vi "TestRoomFGVRequests.vi"() -> (0 "error out":errorcluster, 2 "Pass":bool)   [LabVIEW 2015]
uses:
  TypeDef/RoomsActionEnum.ctl
  LVClasses/Flags/Flags.lvclass
  LVClasses/Room/Room.lvclass
panel:
  out "Add Request 2":string
  out "Read Request 2":string
  out "Remove Request":string
  out "Add Request 1":string
  out "Read Room 3":string
  out "Read Room 1":string
  out "Read Room 2":string
  out "Read Requests 1":string
  in  "FGV Room":i32=102
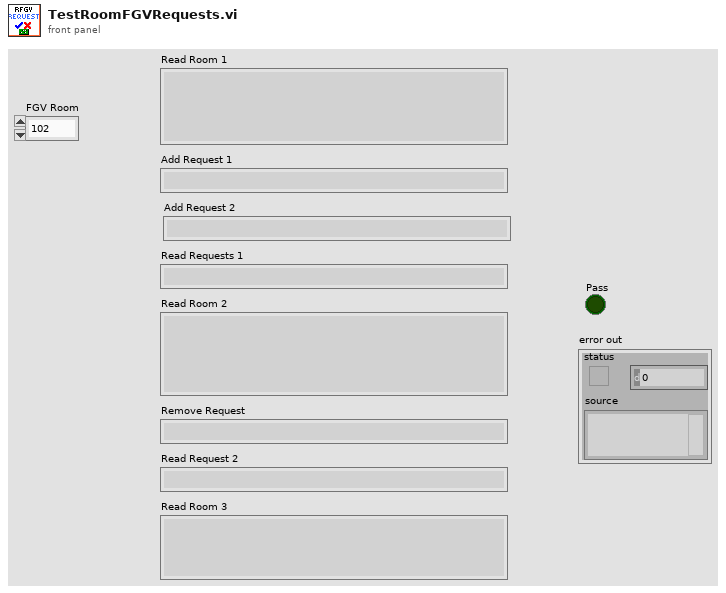
[diagram p1: front panel]
types:
  T1 = typedef "RoomsActionEnum.ctl" = enum16{"Init", "Add Room", "Remove Room", "Read Room", "Read Flag", "Read Flag State", "Write Flag State", "Read Flag Color", "Write Flag Color", "Read Bed Vacant", "Write Bed Vacant", "Read Personnel", "Add Personnel", "Remove Personnel", "Read Requests", "Add Request", "Remove Request", "Read Beacon ID", "Write Beacon ID", "Write Bed URL", "Read Bed URL", "Get Rooms Numbers"}
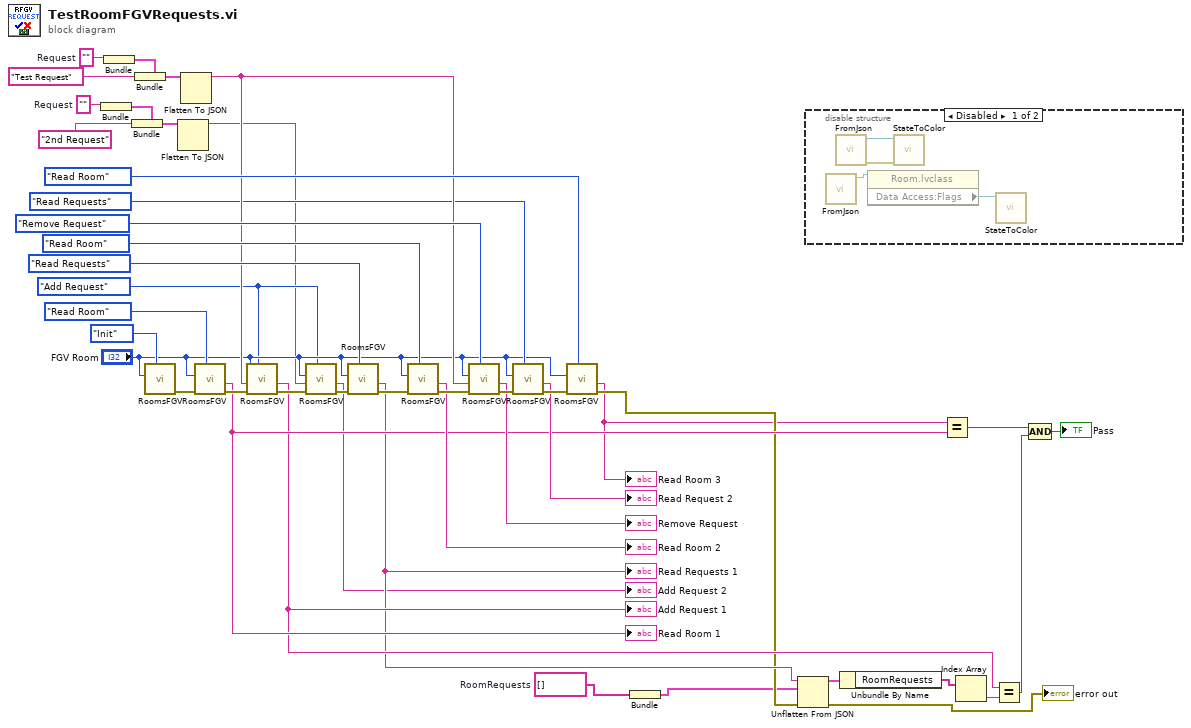
[diagram p0: block diagram]
diagram:
  w8 = ""  # Request
  w5 = string[] []  # RoomRequests
  w34 = ""  # Request
  w12 = RoomsActionEnum."Add Request"
  n1 = Bundle("Request"=w8) -> (w9:cluster{"Request":string})  [unwired: 1 in]
  n2 = Bundle("Request"=w34) -> (w33:cluster{"Request":string})  [unwired: 1 in]
  n3 = Bundle(cluster=w9, "Request"="2nd Request" ("Request 2")) -> (w10:cluster{"Request":string})
  n4 = Bundle(cluster=w33, "Request"="Test Request") -> (w32:cluster{"Request":string})
  n5 = call "RoomsFGV.vi"("Actions"=RoomsActionEnum."Init", "Room"="FGV Room") -> ("error out"=w44:errorcluster)  [unwired: 8 in, 1 out]
  n6 = Flatten To JSON(anything=w10) -> (JSON string=w7:string)  [unwired: 2 in, 1 out]
  n7 = Flatten To JSON(anything=w32) -> (JSON string=w28:string)  [unwired: 2 in, 1 out]
  n8 = call "RoomsFGV.vi"("Actions"=RoomsActionEnum."Read Room", "error in (no error)"=w44, "Room"="FGV Room") -> ("error out"=w43:errorcluster, "Data Out"=w24:string)  [unwired: 7 in]
  "Read Room 1" <- w24
  n9 = call "RoomsFGV.vi"("Actions"=w12, "error in (no error)"=w43, "Data In"=w28, "Room"="FGV Room") -> ("error out"=w35:errorcluster, "Data Out"=w20:string)  [unwired: 6 in]
  "Add Request 1" <- w20
  n10 = call "RoomsFGV.vi"("Actions"=w12, "error in (no error)"=w35, "Data In"=w7, "Room"="FGV Room") -> ("error out"=w14:errorcluster, "Data Out"=→"Add Request 2":string)  [unwired: 6 in]
  n11 = call "RoomsFGV.vi"("Actions"=RoomsActionEnum."Read Requests", "error in (no error)"=w14, "Room"="FGV Room") -> ("error out"=w42:errorcluster, "Data Out"=w19:string)  [unwired: 7 in]
  "Read Requests 1" <- w19
  n12 = call "RoomsFGV.vi"("Actions"=RoomsActionEnum."Read Room", "error in (no error)"=w42, "Room"="FGV Room") -> ("error out"=w38:errorcluster, "Data Out"=→"Read Room 2":string)  [unwired: 7 in]
  n13 = call "RoomsFGV.vi"("Actions"=RoomsActionEnum."Remove Request", "error in (no error)"=w38, "Data In"=w28, "Room"="FGV Room") -> ("error out"=w31:errorcluster, "Data Out"=→"Remove Request":string)  [unwired: 6 in]
  n14 = call "RoomsFGV.vi"("Actions"=RoomsActionEnum."Read Requests", "error in (no error)"=w31, "Room"="FGV Room") -> ("error out"=w30:errorcluster, "Data Out"=→"Read Request 2":string)  [unwired: 7 in]
  n15 = call "RoomsFGV.vi"("Actions"=RoomsActionEnum."Read Room", "error in (no error)"=w30, "Room"="FGV Room") -> ("error out"=w16:errorcluster, "Data Out"=w1:string)  [unwired: 7 in]
  "Read Room 3" <- w1
  n16 = Bundle("RoomRequests"=w5) -> (w4:cluster{"RoomRequests":string[]})  [unwired: 1 in]
  n17 = Unflatten From JSON(JSON string=w19, type and defaults=w4, error in (no error)=w16) -> (value=w3:cluster{"RoomRequests":string[]}, error out=→"error out":errorcluster)  [unwired: 4 in]
  n18 = disable-structure shown="Disabled" {
    frame Disabled {
      n19 = call "FromJson.vi"() -> ("Room out"=w47:refnum<class "Room.lvclass">)  [unwired: 10 in, 1 out]
      n20 = call "FromJson.vi"() -> ("error out"=w49:errorcluster, "Flags out"=w48:refnum<class "Flags.lvclass">)  [unwired: 10 in]
      n21 = property class="Room.lvclass"(reference=w47) -> ("Data Access:Flags"=w46:refnum<class "Flags.lvclass">)  [unwired: 1 in, 2 out]
      n22 = call "StateToColor.vi"("error in (no error)"=w49, "Flags in"=w48) -> ()  [unwired: 7 in, 3 out]
      n23 = call "StateToColor.vi"("Flags in"=w46) -> ()  [unwired: 8 in, 3 out]
    }
    frame Enabled {
    }
  }
  n24 = Unbundle By Name(w3) -> ("RoomRequests"=w2:string[])
  n25 = Equal?(x=w1, y=w24) -> (x = y?=w23:bool)
  n26 = Index Array(array=w2) -> (element=w17:string)  [unwired: 1 in]
  n27 = Equal?(x=w20, y=w17) -> (x = y?=w21:bool)
  n28 = Compound Arithmetic op=AND(w23, w21) -> (→"Pass":bool)
